vi "Method.vi"(4 "Input B":refnum<class "Abs_Numeric.lvclass">, 5 "Input A":T1) -> (1 "Result":T1)   [LabVIEW 2021, in "Subtract_EXT.lvclass"]
uses:
  Subtract_EXT.lvclass
  Abs Type.ctl
  Abs_Types/Extended Float/Abs_Extended Float.lvclass
  Abs_Types/Numeric/Abs_Numeric.lvclass
  C:/Users/Tim/Documents/LabVIEW/2021/Data Classes/Source/Functions/Support/Two Terminal/EXT/AbsFunc_Two Term_EXT.lvclass
  C:/Users/Tim/Documents/LabVIEW/2021/Data Classes/Source/Abs_Types/Extended Float/Abs_Extended Float.lvclass
  Support/Two Terminal/EXT/AbsFunc_Two Term_EXT.lvclass/AbsFunc_Two Term_EXT.ctl
  Support/Two Terminal/EXT/Properties/Write Numeric A.vi
  Support/Two Terminal/EXT/Properties/Write Numeric B.vi
  Subtract_EXT.lvclass/Subtract_EXT.ctl
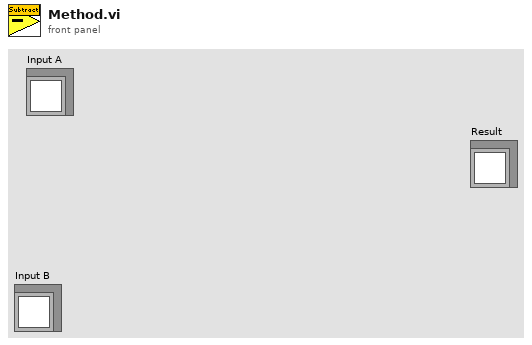
[diagram p1: front panel]
types:
  T1 = typedef "Subtract_EXT.lvclass/Abs Type.ctl" = refnum<class "Abs_Extended Float.lvclass">
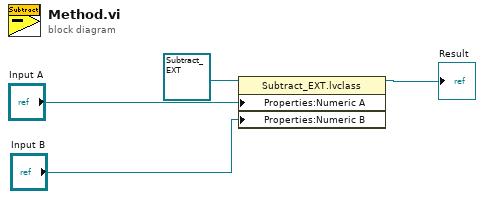
[diagram p0: block diagram]
diagram:
  n1 = property class="Subtract_EXT.lvclass"(reference=refnum<class "Subtract_EXT.lvclass"> refnum ("Subtract_DBL.lvclass"), "Properties:Numeric A"="Input A", "Properties:Numeric B"="Input B") -> (reference out=→"Result":refnum<class "Subtract_EXT.lvclass">)  [unwired: 1 in, 1 out]
